vi "sub_SDR_siso_AWGN_channel.vi"(10 "Channel conf":T1={"Atenuation [dB]"=6.0, "Noise Std. Dev."=0.0, "Initial phase [deg]"=125.0, "Freq. Shift [Hz/Hz]"=0.001} {"Freq. Shift [Hz/Hz]" min=0.0 max=1.0 step=0.0001 format="%0.4f"; "Noise Std. Dev." format="%0.2f"; "Atenuation [dB]" format="%0.2f"}, 11 "Shaped symbols":cdb[](array[numeric])) -> (3 "Array":cdb[](array[numeric]))   [LabVIEW 2012]
uses:
  <vilib>/Analysis/NI_AALBase.lvlib
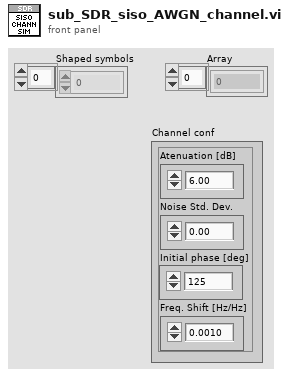
[diagram p1: front panel]
types:
  T1 = cluster{"Atenuation [dB]":dbl, "Noise Std. Dev.":dbl, "Initial phase [deg]":dbl, "Freq. Shift [Hz/Hz]":dbl}
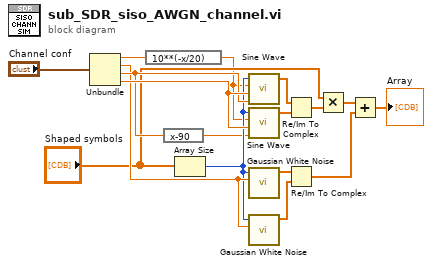
[diagram p0: block diagram]
diagram:
  n1 = Unbundle("Channel conf") -> ("Atenuation [dB]"=w14:dbl, "Noise Std. Dev."=w15:dbl, "Initial phase [deg]"=w16:dbl, "Freq. Shift [Hz/Hz]"=w17:dbl)
  n2 = expression code="10**(-x/20)"(w14) -> (w6:dbl)
  n3 = expression code="x-90"(w16) -> (w5:dbl)
  n4 = Array Size(array="Shaped symbols") -> (size(s)=w7:i32)
  n5 = call <vilib>:"Sine Wave.vi"("samples"=w7, "amplitude"=w6, "frequency"=w17, "phase in"=w16) -> ("sine wave"=w8:dbl[])  [unwired: 1 in, 2 out]
  n6 = call <vilib>:"Sine Wave.vi"("samples"=w7, "amplitude"=w6, "frequency"=w17, "phase in"=w5) -> ("sine wave"=w9:dbl[])  [unwired: 1 in, 2 out]
  n7 = call <vilib>:"Gaussian White Noise.vi"("standard deviation"=w15, "samples"=w7) -> ("Gaussian noise pattern"=w2:dbl[])  [unwired: 8 in, 1 out]
  n8 = call <vilib>:"Gaussian White Noise.vi"("standard deviation"=w15, "samples"=w7) -> ("Gaussian noise pattern"=w3:dbl[])  [unwired: 8 in, 1 out]
  n9 = Re/Im To Complex(1:w9, 2:w8) -> (0:w10:cdb[])
  n10 = Re/Im To Complex(1:w3, 2:w2) -> (0:w4:cdb[])
  n11 = Multiply(x="Shaped symbols", y=w10) -> (x*y=w12:cdb[])
  n12 = Add(x=w12, y=w4) -> (x+y=→"Array":cdb[])
